vi "CreateStructure.vi"(6 "UID":i32, 7 "PythonConverter in":refnum<class "PythonBDConverter.lvclass">, 8 "error in":errorcluster, 11 "VI Interpreter in":refnum<class "VI Interpreter.lvclass">) -> (0 "error out":errorcluster, 3 "VI Interpreter out":refnum<class "VI Interpreter.lvclass">, 5 "PythonConverter out":refnum<class "PythonBDConverter.lvclass">)   [LabVIEW 2014, in "PythonBDConverter.lvclass"]
uses:
  PythonBDConverter.lvclass
  VI Interpreter/Classes/VI Interpreter/VI Interpreter.lvclass
  VI Interpreter/Classes/Structure/Structure.lvclass
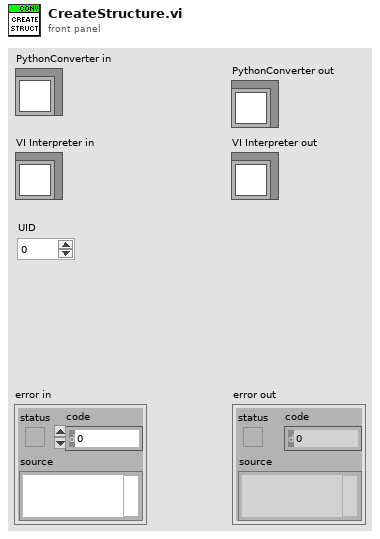
[diagram p1: front panel]
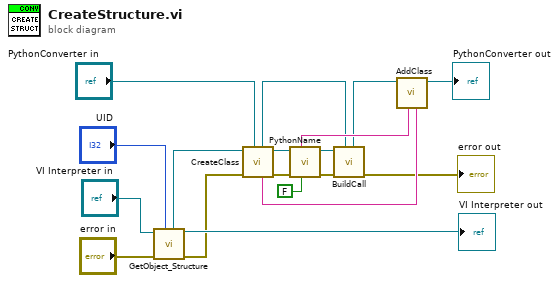
[diagram p0: block diagram]
diagram:
  n1 = call "GetObject_Structure.vi"("UID"="UID", "error in"="error in", "VI Interpreter in"="VI Interpreter in") -> ("error out"=w8:errorcluster, "VI Interpreter out"=→"VI Interpreter out":refnum<class "VI Interpreter.lvclass">, "structure"=w11:refnum<class "Structure.lvclass">)  [unwired: 3 in, 1 out]
  n2 = call-dynamic "CreateClass.vi"("PythonConverter in"="PythonConverter in", "error in"=w8, "GObject in"=w11) -> ("error out"=w15:errorcluster, "GObject out"=w16:refnum<class "Structure.lvclass">, "class"=w12:string, "PythonConverter out"=w4:refnum<class "PythonBDConverter.lvclass">)  [unwired: 5 in]
  n3 = call-dynamic "PythonName.vi"("add self"=FALSE, "error in"=w15, "Node in"=w16) -> ("error out"=w5:errorcluster, "Node out"=w6:refnum<class "Structure.lvclass">, "UID"=w7:string)  [unwired: 5 in, 1 out]
  n4 = call-dynamic "BuildCall.vi"("PythonConverter in"=w4, "error in"=w5, "Structure in"=w6) -> ("error out"=→"error out":errorcluster, "PythonConverter out"=w3:refnum<class "PythonBDConverter.lvclass">)  [unwired: 6 in, 1 out]
  n5 = call "AddClass.vi"("definition"=w12, "name"=w7, "PythonConverter in"=w3) -> ("PythonConverter out"=→"PythonConverter out":refnum<class "PythonBDConverter.lvclass">)  [unwired: 5 in, 1 out]
